vi "Run Test.vi"(8 "error in (no error)":errorcluster, 11 "Measurement in":refnum<class "Efficiency Test.lvclass">) -> (0 "error out":errorcluster, 1 "Positions":i32[](array[numeric]), 2 "Tests Passed":bool[](array[boolean]), 3 "Measurement out":refnum<class "Efficiency Test.lvclass">, 5 "Fail Codes":string[](array[string]))   [LabVIEW 2015, in "Efficiency Test.lvclass"]
uses:
  Efficiency Test.lvclass
  Test Class/Test Class.lvclass
  Classes/Application/Class/Application.lvclass
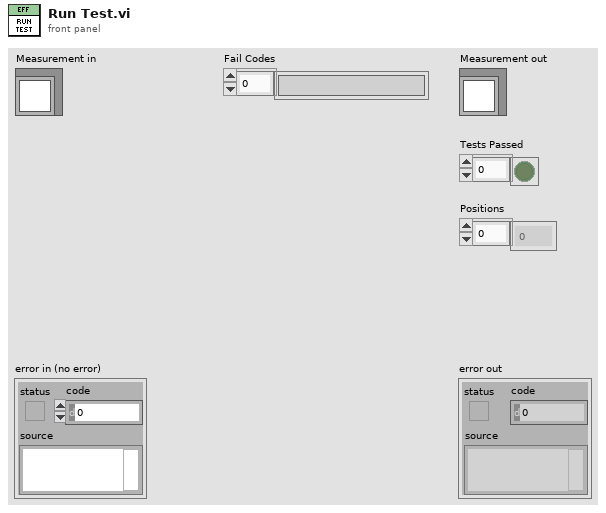
[diagram p1: front panel]
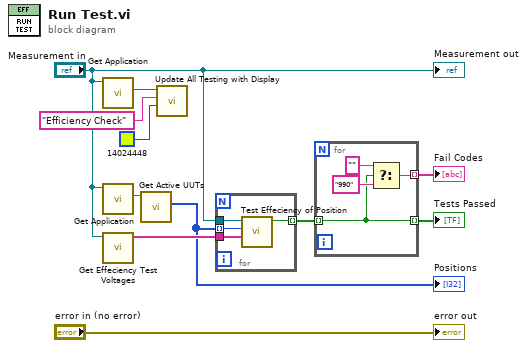
[diagram p0: block diagram]
diagram:
  n1 = call "Get Application.vi"("Test Class in"="Measurement in") -> ("Application.lvlib:Application.lvclass"=w8:refnum<class "Application.lvclass">)  [unwired: 9 in, 1 out]
  n2 = call "Get Application.vi"("Test Class in"="Measurement in") -> ("Application.lvlib:Application.lvclass"=w4:refnum<class "Application.lvclass">)  [unwired: 9 in, 1 out]
  n3 = call "Get Effeciency Test Voltages.vi"("Efficiency Test in"="Measurement in") -> ("Test Voltages"=w3:string[])  [unwired: 10 in]
  n4 = call "Get Active UUTs.vi"("Application in"=w4) -> ("Active Positions"=w1:u32[])  [unwired: 8 in, 2 out]
  "Positions" <- w1
  n5 = call "Update All Testing with Display.vi"("BG Color"=u32 14024448, "Message ('')"="Efficiency Check", "Application in"=w8) -> ()  [unwired: 7 in, 2 out]
  n6 = for {
    tunnel: "Measurement in" -> [w15]
    tunnel: w1 -> [w14] mode=indexing
    tunnel: w3 -> [w13]
    tunnel: [w12] -> w2 mode=indexing
    n7 = call "Test Effeciency of Position.vi"("Test Voltages"=w13, "Position"=w14, "Efficiency Test in"=w15) -> ("Effeciency Passed"=w12:bool)  [unwired: 8 in]
  }
  n8 = for {
    tunnel: [w18] -> w11 mode=indexing
    tunnel: [w16] -> w7 mode=indexing
    tunnel: w2 -> [w16] mode=indexing
    n9 = Select(t="", s=w16, f="990") -> (s? t:f=w18:string)
  }
  "Tests Passed" <- w7
  "Fail Codes" <- w11
  "error out" <- "error in (no error)"
  "Measurement out" <- "Measurement in"
